vi "Configure Channel.vi"(8 "error in (no error)":errorcluster, 10 "Channel Setting":T1={"Channel Name (0: Channel 1)"=0, "Coupling (1: DC)"=1, "Vertical Offset (0.0)"=0.0, "Vertical Range (40.0 V)"=40.0, "Probe Attenuation (1.0)"=1.0, "Enable Channel (T: Enable)"=TRUE, "Impedance (0: 1 MOhm)"=0, "Vertical Scale (5.0 V)"=5.0, "Vertical Setting (1: Vertical Range)"=1} {"Vertical Setting (1: Vertical Range)" items=["Vertical Scale", "Vertical Range"]; "Impedance (0: 1 MOhm)" items=["1 MOhm", "50 Ohm"]; "Coupling (1: DC)" items=["AC", "DC"]; "Channel Name (0: Channel 1)" items=["Channel 1", "Channel 2", "Channel 3", "Channel 4"]}, 11 "Agilent 3054A in":refnum<class "Agilent 3054A.lvclass">) -> (0 "error out":errorcluster, 3 "Agilent 3054A out":refnum<class "Agilent 3054A.lvclass">)   [LabVIEW 2016, in "Oscilloscope.lvlib" / "Agilent 3054A.lvclass"]
uses:
  Agilent 3054A.lvclass
  Agilent 3054A.lvclass/Agilent 3054A.ctl
  <instrlib>/Agilent 2000 3000 X-Series/Agilent 2000 3000 X-Series.lvlib
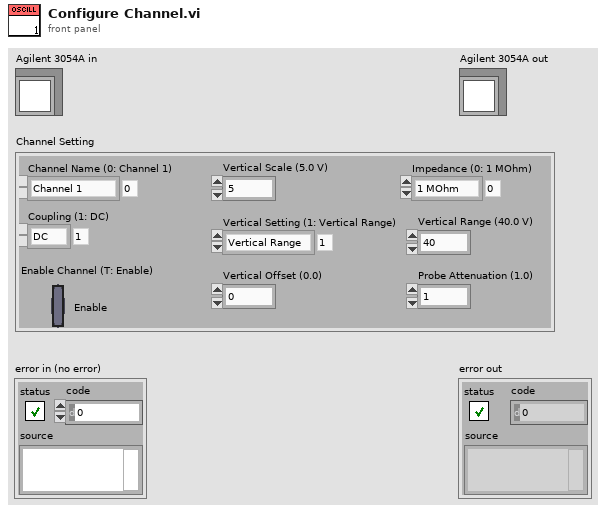
[diagram p1: front panel]
types:
  T1 = cluster{"Channel Name (0: Channel 1)":i32, "Coupling (1: DC)":i32, "Vertical Offset (0.0)":dbl, "Vertical Range (40.0 V)":dbl, "Probe Attenuation (1.0)":dbl, "Enable Channel (T: Enable)":bool, "Impedance (0: 1 MOhm)":i32, "Vertical Scale (5.0 V)":dbl, "Vertical Setting (1: Vertical Range)":i32}
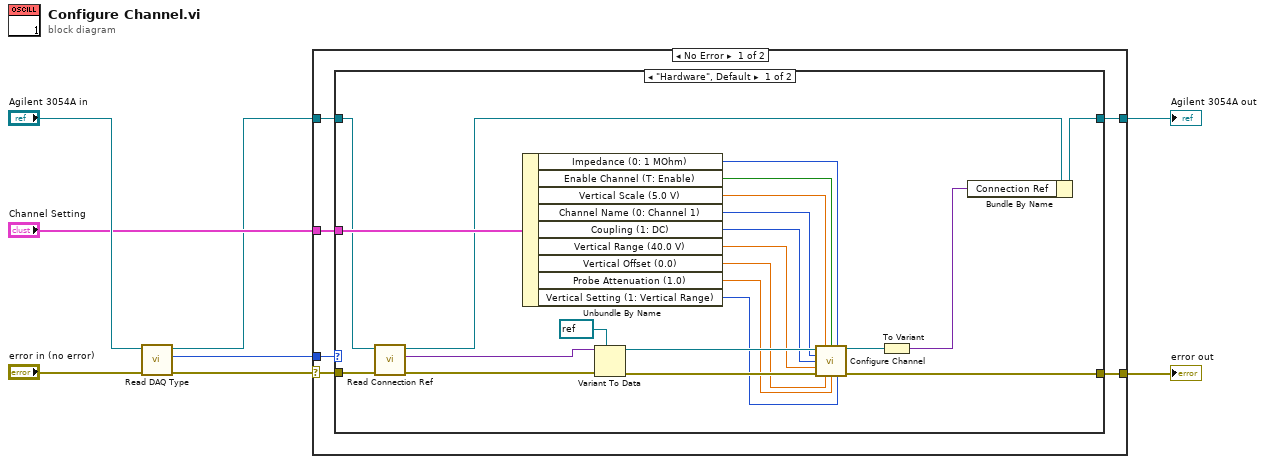
[diagram p0: block diagram]
diagram:
  n1 = call-dynamic "Read DAQ Type.vi"("error in (no error)"="error in (no error)", "Agilent 3054A in"="Agilent 3054A in") -> ("error out"=w7:errorcluster, "DAQ Type"=w6:enum16{"Hardware", "Simulation"}, "Agilent 3054A out"=w1:refnum<class "Agilent 3054A.lvclass">)  [unwired: 7 in]
  n2 = case shown="No Error" w7 {
    selector: w7 -> [w12 w39]
    tunnel: w6 -> [w14 _]
    tunnel: w1 -> [w13 w40]
    tunnel: "Channel Setting" -> [w11 _]
    tunnel: [w10 w40] -> w3
    tunnel: [w9 w39] -> w2
    frame No Error {
      n3 = case shown="\"Hardware\", Default" w14 {
        tunnel: w13 -> [w16 w38]
        tunnel: w12 -> [w36 w37]
        tunnel: w11 -> [w30 _]
        tunnel: [w20 w38] -> w10
        tunnel: [w21 w37] -> w9
        frame "Hardware", Default {
          n4 = call-dynamic "Read Connection Ref.vi"("error in (no error)"=w36, "Agilent 3054A in"=w16) -> ("error out"=w35:errorcluster, "Connection Ref"=w34:variant, "Agilent 3054A out"=w15:refnum<class "Agilent 3054A.lvclass">)  [unwired: 7 in]
          n5 = Unbundle By Name(w30) -> ("Impedance (0: 1 MOhm)"=w29:i32, "Enable Channel (T: Enable)"=w28:bool, "Vertical Scale (5.0 V)"=w27:dbl, "Channel Name (0: Channel 1)"=w26:i32, "Coupling (1: DC)"=w25:i32, "Vertical Range (40.0 V)"=w24:dbl, "Vertical Offset (0.0)"=w23:dbl, "Probe Attenuation (1.0)"=w22:dbl, "Vertical Setting (1: Vertical Range)"=w18:i32)
          n6 = Variant To Data(error in=w35, type=refnum<visa-resource-name> refnum ("VISA resource name"), Variant=w34) -> (data=w31:refnum<visa-resource-name>, error out=w32:errorcluster)
          n7 = call <instrlib>:"Configure Channel.vi"("VISA resource name"=w31, "Vertical Scale (5.0 V)"=w27, "Enable Channel (T: Enable)"=w28, "Impedance (0: 1 MOhm)"=w29, "Channel Name (0: Channel 1)"=w26, "Coupling (1: DC)"=w25, "Vertical Range (40.0 V)"=w24, "error in (no error)"=w32, "Vertical Offset (0.0)"=w23, "Probe Attenuation (1.0)"=w22, "Vertical Setting (1: Vertical Range)"=w18) -> ("VISA resource name out"=w19:refnum<visa-resource-name>, "error out"=w21:errorcluster)  [unwired: 3 in]
          n8 = To Variant(anything=w19) -> (Variant=w17:variant)
          n9 = Bundle By Name(cluster=w15, "Connection Ref"=w17) -> (w20:refnum<class "Agilent 3054A.lvclass">)
        }
        frame "Simulation" {
        }
      }
    }
    frame Error {
    }
  }
  "error out" <- w2
  "Agilent 3054A out" <- w3
